vi "SpecSave.vi"(6 "Save All Acq Counts":bool, 8 "DeviceName":string, 9 "AllAcqCounts":dbl[][](array[numeric]), 10 "Path":path, 11 "SelectedShotArray":dbl[][](array[numeric])) -> ()   [LabVIEW 2020, in "HamamatsuSpectrometerDAQ.lvclass"]
uses:
  HamamatsuSpectrometerDAQ.lvclass
panel:
  out "x-y":u32
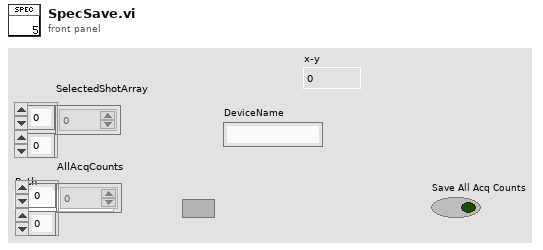
[diagram p1: front panel]
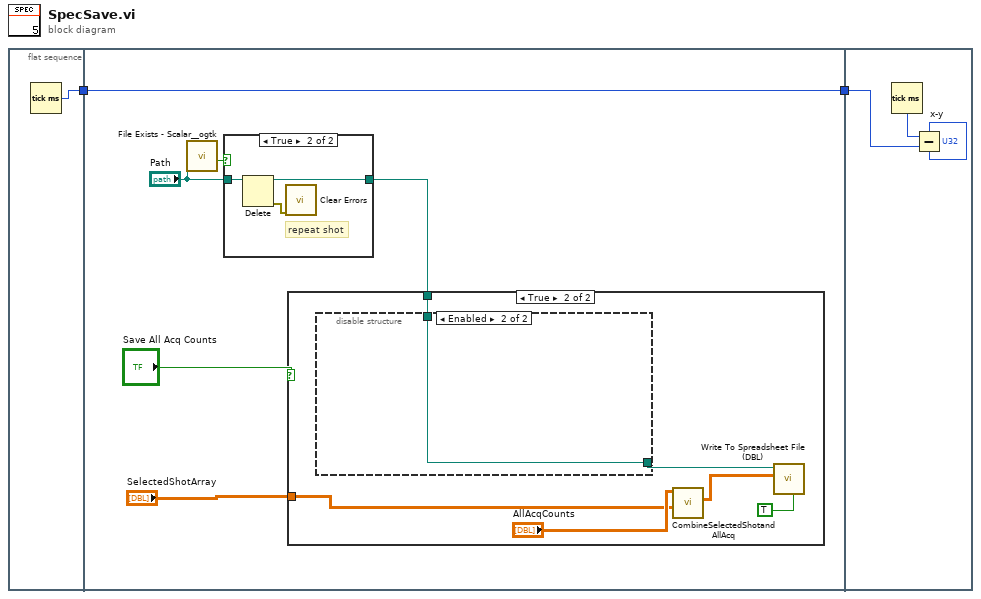
[diagram p0: block diagram]
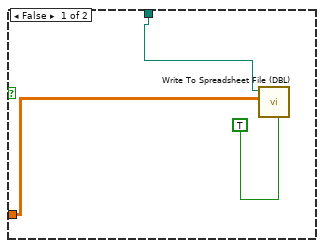
[diagram p2: hidden frame]
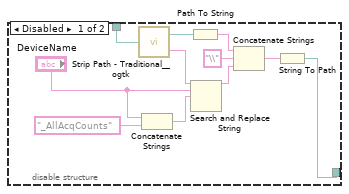
[diagram p3: hidden frame]
diagram:
  n1 = flat-sequence {
    tunnel: [w3] -> w1
    tunnel: [w7] -> w2
    tunnel: w1 -> [w7]
    tunnel: w2 -> [w36]
    frame #0 {
      n2 = Tick Count (ms)() -> (millisecond timer value=w3:u32)
    }
    frame #1 {
      n3 = call "File Exists - Scalar__ogtk.vi"("file path"="Path") -> ("exists"=w9:bool)  [unwired: 6 in, 1 out]
      n4 = case shown="True" w9 {
        tunnel: "Path" -> [w31 w34]
        tunnel: [w31 w32] -> w5
        frame False {
        }
        frame True {
          # "repeat shot"
          n5 = Delete(path (use dialog)=w34) -> (deleted path=w32:path, error out=w33:errorcluster)  [unwired: 4 in, 1 out]
          n6 = call "Clear Errors.vi"("error in (no error)"=w33) -> ()  [unwired: 5 in, 2 out]
        }
      }
      n7 = case shown="True" "Save All Acq Counts" {
        tunnel: w5 -> [w11 w17]
        tunnel: "SelectedShotArray" -> [w10 w14]
        frame False {
          n8 = call "Write To Spreadsheet File (DBL).vi"("transpose? (no:F)"=TRUE, "2D data"=w10, "file path (dialog if empty)"=w11) -> ()  [unwired: 5 in, 1 out]
        }
        frame True {
          n9 = disable-structure shown="Enabled" {
            disable-tunnel: w17 -> [w29 w30]
            disable-tunnel: [w19 w30] -> w16
            frame Disabled {
              n10 = call "Strip Path - Traditional__ogtk.vi"("path"=w29) -> ("stripped path"=w24:path, "name"=w28:string)
              n11 = Concatenate Strings("DeviceName", "_AllAcqCounts" ("replace string (\"\")")) -> (w25:string)
              n12 = Path To String(path=w24) -> (string=w21:string)
              n13 = Search and Replace String(input string=w28, search string="DeviceName", replace string=w25) -> (result string=w20:string)  [unwired: 5 in, 3 out]
              n14 = Concatenate Strings(w21, "\\" ("string"), w20) -> (w23:string)
              n15 = String To Path(string=w23) -> (path=w19:path)
            }
            frame Enabled {
            }
          }
          n16 = call "CombineSelectedShotandAllAcq.vi"("Selected Shot Array"=w14, "AllAcq Array"="AllAcqCounts") -> ("Combined Array"=w13:dbl[][])  [unwired: 9 in]
          n17 = call "Write To Spreadsheet File (DBL).vi"("transpose? (no:F)"=TRUE, "2D data"=w13, "file path (dialog if empty)"=w16) -> ()  [unwired: 5 in, 1 out]
        }
      }
    }
    frame #2 {
      n18 = Tick Count (ms)() -> (millisecond timer value=w37:u32)
      n19 = Subtract(x=w37, y=w36) -> (x-y=→"x-y":u32)
    }
  }
